vi "SaveMultiToolMeasurementDataToFileSubVI.vi"(1 "Array of Time for Measurement":string[](array[string]), 2 "NDI Tool":string, 4 "Array - Transformations of Tool 2":T1(array[cluster]), 5 "Array - Transformations of Tool 1":T1(array[cluster]), 6 "error in (no error)":errorcluster, 7 "Object number":string, 8 "Output Directory":path, 9 "VISA Refnum in":refnum<visa-resource-name>) -> (0 "error out":errorcluster, 3 "VISA Refnum out":refnum<visa-resource-name>)   [LabVIEW 2013]
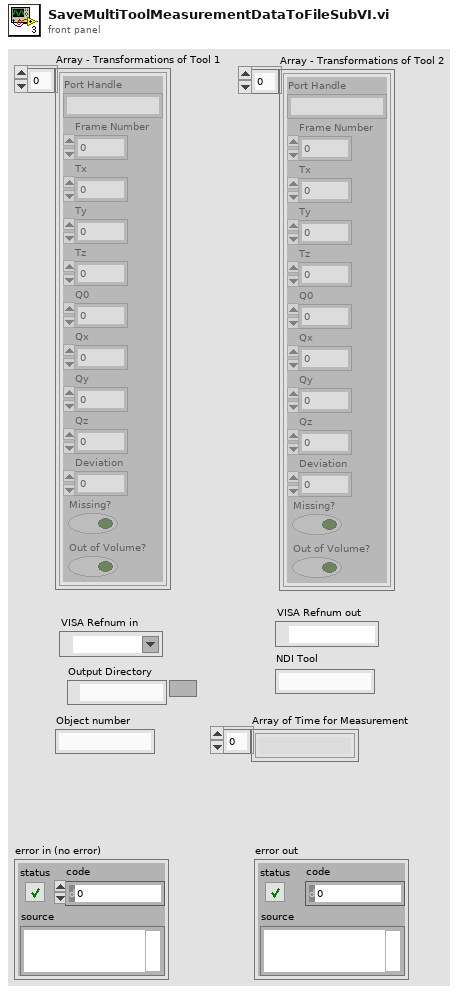
[diagram p1: front panel]
types:
  T1 = cluster{"Port Handle":string, "Frame Number":u32, "Tx":dbl, "Ty":dbl, "Tz":dbl, "Q0":dbl, "Qx":dbl, "Qy":dbl, "Qz":dbl, "Deviation":dbl, "Missing?":bool, "Out of Volume?":bool}[]
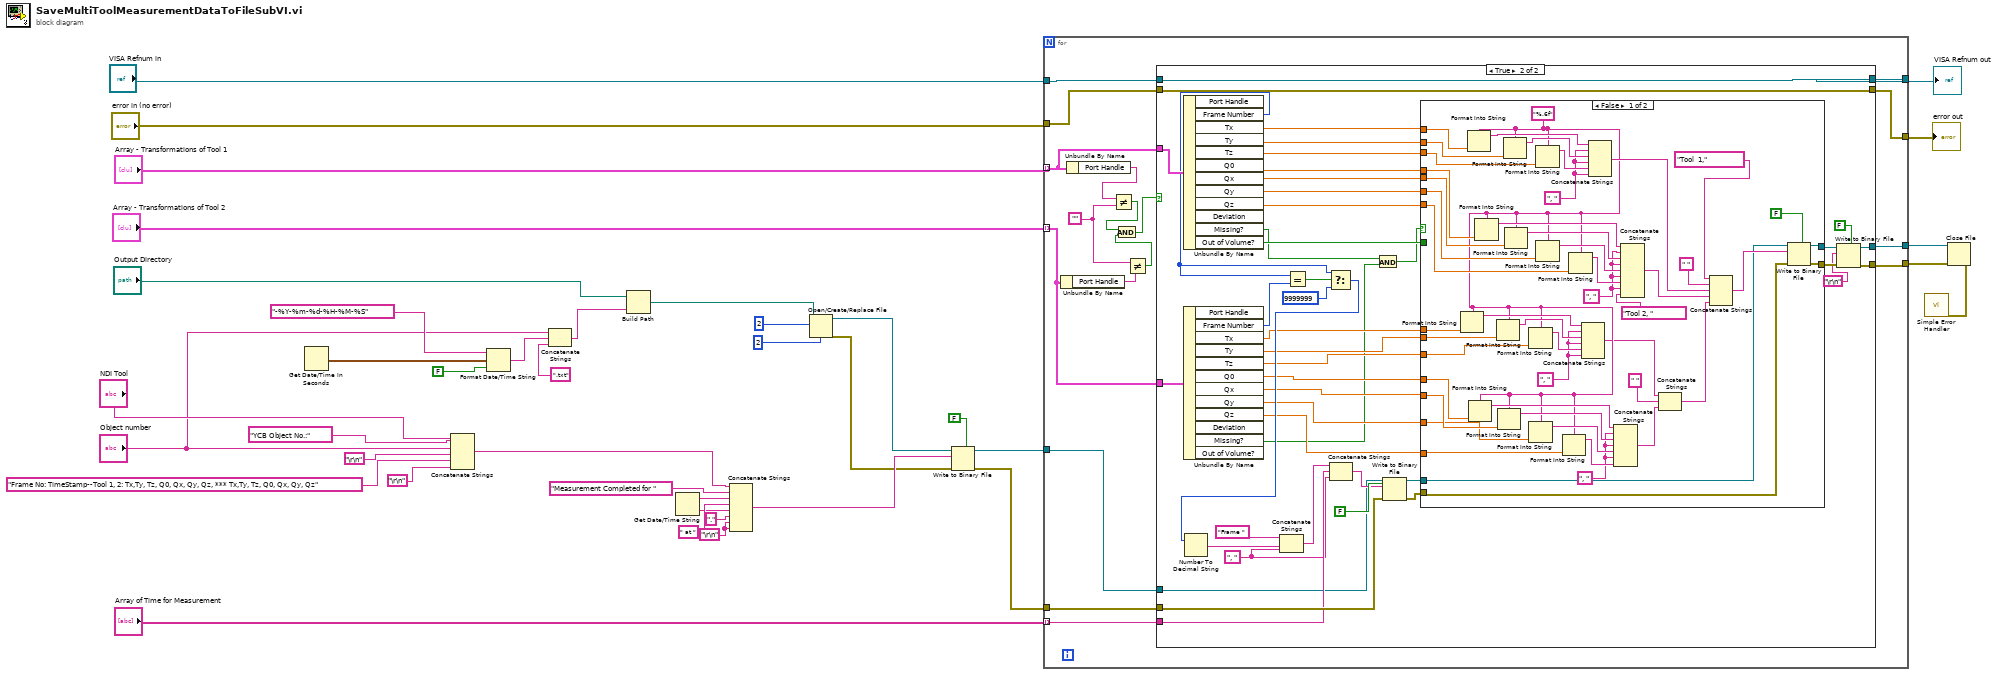
[diagram p0: block diagram]
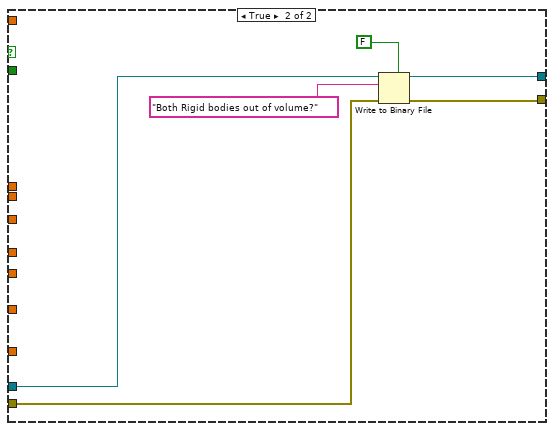
[diagram p3: hidden frame]
diagram:
  w30 = "\r\n"
  n1 = Get Date/Time In Seconds() -> (seconds since 1Jan1904=w23:timestamp)
  n2 = Concatenate Strings("NDI Tool", "YCB Object No.:", "Object number", "\r\n", "Frame No: TimeStamp--Tool 1, 2: Tx,Ty, Tz, Q0, Qx, Qy, Qz, *** Tx,Ty, Tz, Q0, Qx, Qy, Qz", "\r\n") -> (w9:string)
  n3 = Format Date/Time String(time format string (%c)="-%Y-%m-%d-%H-%M-%S", seconds (now)=w23, UTC format=FALSE) -> (date/time string=w26:string)
  n4 = Concatenate Strings("Object number", w26, ".txt") -> (w25:string)
  n5 = Build Path(base path="Output Directory", name or relative path=w25) -> (appended path=w24:path)
  n6 = Get Date/Time String() -> (date string=w35:string, time string=w33:string)  [unwired: 3 in]
  n7 = Concatenate Strings(w9, "Measurement Completed for ", w35, " at ", w33, "." ("string"), w30, w30) -> (w32:string)
  n8 = Open/Create/Replace File(file path (use dialog)=w24, operation (0:open)=i8 2, access (0:read/write)=i8 2) -> (refnum out=w16:refnum<file>, error out=w17:errorcluster)  [unwired: 3 in, 1 out]
  n9 = Write to Binary File(file (use dialog)=w16, data=w32, error in=w17, 5:FALSE ("prepend array or string size? (T)")) -> (refnum out=w14:refnum<file>, error out=w15:errorcluster)  [unwired: 2 in, 1 out]
  n10 = for {
    tunnel: w14 -> [w56]
    tunnel: [w54] -> w12
    tunnel: "Array - Transformations of Tool 1" -> [w51] mode=indexing
    tunnel: "Array of Time for Measurement" -> [w52] mode=indexing
    tunnel: "VISA Refnum in" -> [w50]
    tunnel: "error in (no error)" -> [w47]
    tunnel: [w49] -> w10
    tunnel: [w48] -> w8
    tunnel: w15 -> [w55]
    tunnel: [w53] -> w13
    tunnel: "Array - Transformations of Tool 2" -> [w40] mode=indexing
    w45 = ""
    n11 = Unbundle By Name(w40) -> ("Port Handle"=w46:string)
    n12 = Unbundle By Name(w51) -> ("Port Handle"=w43:string)
    n13 = Not Equal?(x=w43, y=w45) -> (x != y?=w42:bool)
    n14 = Not Equal?(x=w45, y=w46) -> (x != y?=w44:bool)
    n15 = And(x=w42, y=w44) -> (x .and. y?=w41:bool)
    n16 = case shown="True" w41 {
      tunnel: w56 -> [w60 w79]
      tunnel: w55 -> [w59 w104]
      tunnel: [w60 w98] -> w54
      tunnel: [w59 w97] -> w53
      tunnel: w52 -> [_ w85]
      tunnel: w51 -> [_ w88]
      tunnel: w50 -> [w58 w82]
      tunnel: w47 -> [w57 w81]
      tunnel: [w58 w82] -> w49
      tunnel: [w57 w81] -> w48
      tunnel: w40 -> [_ w78]
      frame False {
      }
      frame True {
        w61 = ", " ("string")
        n17 = Unbundle By Name(w88) -> ("Frame Number"=w74:u32, "Tx"=w101:dbl, "Ty"=w100:dbl, "Tz"=w80:dbl, "Q0"=w93:dbl, "Qx"=w92:dbl, "Qy"=w91:dbl, "Qz"=w90:dbl, "Missing?"=w63:bool, "Out of Volume?"=w96:bool)  [unwired: 2 out]
        n18 = Unbundle By Name(w78) -> ("Frame Number"=w76:u32, "Tx"=w71:dbl, "Ty"=w70:dbl, "Tz"=w69:dbl, "Q0"=w68:dbl, "Qx"=w67:dbl, "Qy"=w66:dbl, "Qz"=w65:dbl, "Missing?"=w62:bool)  [unwired: 3 out]
        n19 = Equal?(x=w74, y=w76) -> (x = y?=w75:bool)
        n20 = Select(t=w74, s=w75, f=9999999) -> (s? t:f=w72:u32)
        n21 = Number To Decimal String(number=w72) -> (decimal integer string=w77:string)  [unwired: 1 in]
        n22 = Concatenate Strings("Frame ", w77, w61) -> (w86:string)
        n23 = Concatenate Strings(w86, w85, w61) -> (w87:string)
        n24 = And(x=w63, y=w62) -> (x .and. y?=w64:bool)
        n25 = Write to Binary File(file (use dialog)=w79, data=w87, error in=w104, 5:FALSE ("prepend array or string size? (T)")) -> (refnum out=w103:refnum<file>, error out=w102:errorcluster)  [unwired: 2 in, 1 out]
        n26 = case shown="False" w64 {
          tunnel: w103 -> [w144 w154]
          tunnel: w102 -> [w150 w155]
          tunnel: [w151 w158] -> w99
          tunnel: w101 -> [w152 _]
          tunnel: w100 -> [w142 _]
          tunnel: w96 -> [_ _]
          tunnel: w93 -> [w148 _]
          tunnel: w92 -> [w147 _]
          tunnel: w91 -> [w136 _]
          tunnel: w90 -> [w135 _]
          tunnel: [w145 w157] -> w83
          tunnel: w80 -> [w141 _]
          tunnel: w71 -> [w113 _]
          tunnel: w70 -> [w112 _]
          tunnel: w69 -> [w111 _]
          tunnel: w68 -> [w110 _]
          tunnel: w67 -> [w109 _]
          tunnel: w66 -> [w108 _]
          tunnel: w65 -> [w107 _]
          frame False {
            w118 = ", " ("string")
            w123 = ", " ("string")
            w115 = ", " ("string")
            w137 = ", " ("string")
            w117 = "%.6f" ("format string")
            n27 = Format Into String(format string=w117, w113) -> (resulting string=w126:string)  [unwired: 2 in, 1 out]
            n28 = Format Into String(format string=w117, w152) -> (resulting string=w140:string)  [unwired: 2 in, 1 out]
            n29 = Format Into String(format string=w117, w110) -> (resulting string=w122:string)  [unwired: 2 in, 1 out]
            n30 = Format Into String(format string=w117, w148) -> (resulting string=w134:string)  [unwired: 2 in, 1 out]
            n31 = Format Into String(format string=w117, w112) -> (resulting string=w125:string)  [unwired: 2 in, 1 out]
            n32 = Format Into String(format string=w117, w109) -> (resulting string=w121:string)  [unwired: 2 in, 1 out]
            n33 = Format Into String(format string=w117, w142) -> (resulting string=w139:string)  [unwired: 2 in, 1 out]
            n34 = Format Into String(format string=w117, w147) -> (resulting string=w133:string)  [unwired: 2 in, 1 out]
            n35 = Format Into String(format string=w117, w111) -> (resulting string=w124:string)  [unwired: 2 in, 1 out]
            n36 = Format Into String(format string=w117, w108) -> (resulting string=w120:string)  [unwired: 2 in, 1 out]
            n37 = Format Into String(format string=w117, w141) -> (resulting string=w138:string)  [unwired: 2 in, 1 out]
            n38 = Format Into String(format string=w117, w136) -> (resulting string=w132:string)  [unwired: 2 in, 1 out]
            n39 = Format Into String(format string=w117, w107) -> (resulting string=w119:string)  [unwired: 2 in, 1 out]
            n40 = Format Into String(format string=w117, w135) -> (resulting string=w131:string)  [unwired: 2 in, 1 out]
            n41 = Concatenate Strings(w126, w123, w125, w123, w124, w123) -> (w116:string)
            n42 = Concatenate Strings(w140, w137, w139, w137, w138, w137) -> (w129:string)
            n43 = Concatenate Strings(w122, w118, w121, w118, w120, w118, w119) -> (w106:string)
            n44 = Concatenate Strings(w134, w115, w133, w115, w132, w115, w131, w115, "Tool 2, " ("string")) -> (w130:string)
            n45 = Concatenate Strings(w116, " " ("string"), w106) -> (w105:string)
            n46 = Concatenate Strings("Tool  1,", " " ("string"), w129, w130, w105) -> (w146:string)
            n47 = Write to Binary File(file (use dialog)=w144, data=w146, error in=w150, 5:FALSE ("prepend array or string size? (T)")) -> (refnum out=w145:refnum<file>, error out=w151:errorcluster)  [unwired: 2 in, 1 out]
          }
          frame True {
            n48 = Write to Binary File(file (use dialog)=w154, data="Both Rigid bodies out of volume?", error in=w155, 5:FALSE ("prepend array or string size? (T)")) -> (refnum out=w157:refnum<file>, error out=w158:errorcluster)  [unwired: 2 in, 1 out]
          }
        }
        n49 = Write to Binary File(file (use dialog)=w83, data="\r\n", error in=w99, 5:FALSE ("prepend array or string size? (T)")) -> (refnum out=w98:refnum<file>, error out=w97:errorcluster)  [unwired: 2 in, 1 out]
      }
    }
  }
  "VISA Refnum out" <- w10
  "error out" <- w8
  n50 = Close File(refnum=w12, error in=w13) -> (error out=w29:errorcluster)  [unwired: 1 out]
  n51 = call <vilib>:"Simple Error Handler.vi"("error in (no error)"=w29) -> ()  [unwired: 4 in, 5 out]
